vi "Measured Data (B).vi"(0 "LoadProcedure":refnum<k24>, 5 "error in (no error)":errorcluster) -> (14 "Value X":dbl[](array[numeric]), 15 "Value Y":dbl[](array[numeric]), 16 "Signal X sel":string(combo)="SetpointApplied", 17 "XY Graph":cluster{"Values":dbl[], "Values":dbl[]}(graph), 18 "Signal Y sel":string(combo)="EI_0.CalcCurrent", 19 "error out":errorcluster)   [LabVIEW 2011]
doc: "View the measured data from the procedure. The command and the command parameter of the procedure are selected with constants (basic version)."
uses:
  C:/Program Files/Metrohm Autolab/Autolab SDK 1.10/EcoChemie.Autolab.Sdk.dll
  EcoChemie.Autolab.Sdk.dll
  C:/Program Files/Metrohm Autolab/Autolab SDK 1.10/EcoChemie100.dll
  EcoChemie100.dll
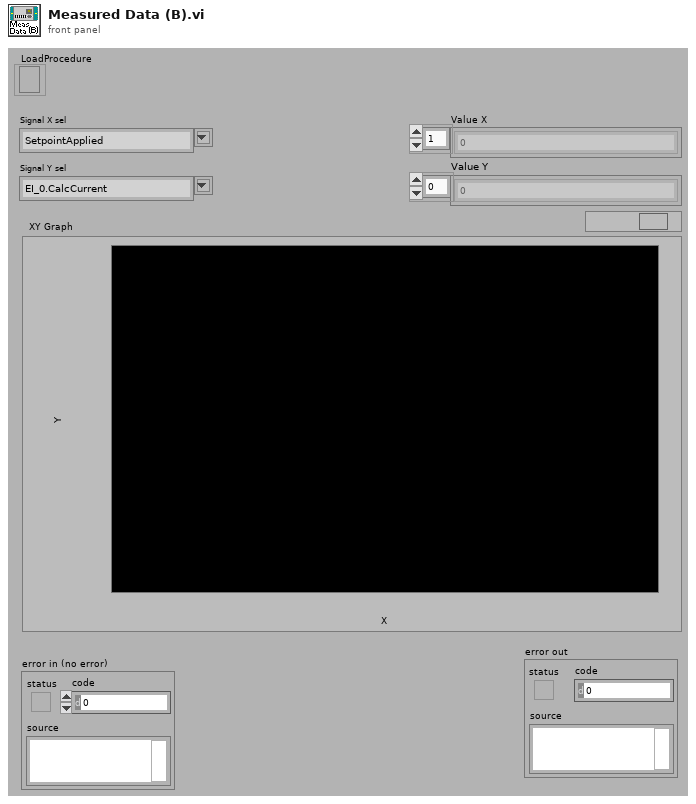
[diagram p1: front panel]
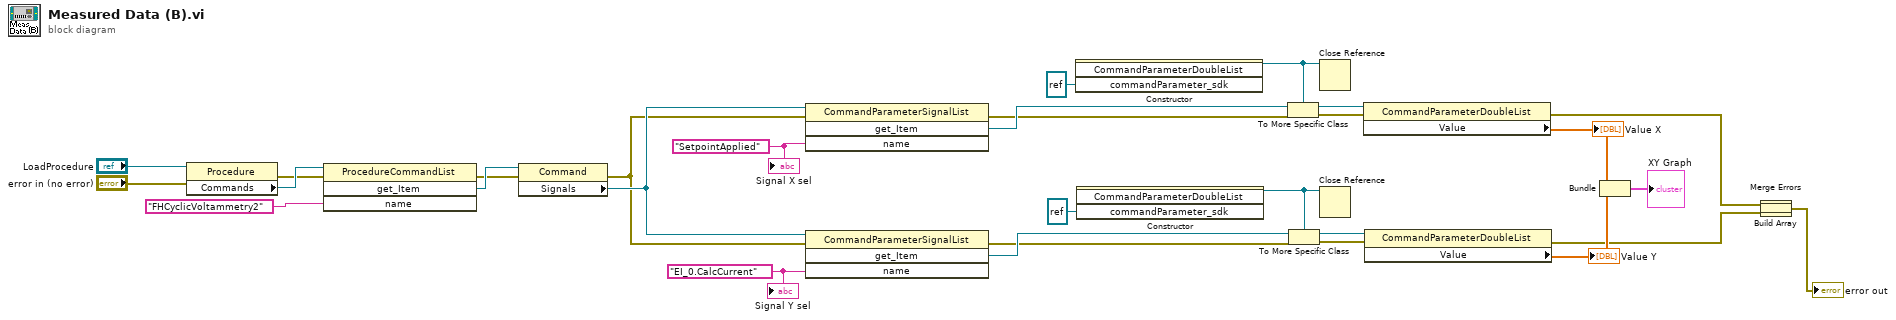
[diagram p0: block diagram]
diagram:
  w25 = "EI_0.CalcCurrent" ("Signal Y sel")
  w22 = "SetpointApplied" ("Signal X sel")
  n1 = property class="Procedure"(reference="LoadProcedure", error in="error in (no error)") -> (error out=w9:errorcluster, "Commands"=w10:refnum<k24>)  [unwired: 1 out]
  n2 = invoke class="ProcedureCommandList" method="get_Item"(reference=w10, error in=w9, "name"="FHCyclicVoltammetry2" ("ProcedureCommandList 2")) -> (error out=w6:errorcluster, "get_Item"=w7:refnum<k24>)  [unwired: 1 in, 2 out]
  n3 = property class="Command"(reference=w7, error in=w6) -> (error out=w12:errorcluster, "Signals"=w13:refnum<k24>)  [unwired: 1 out]
  n4 = invoke class="CommandParameterSignalList" method="get_Item"(reference=w13, error in=w12, "name"=w22) -> (error out=w18:errorcluster, "get_Item"=w19:refnum<k24>)  [unwired: 1 in, 2 out]
  n5 = invoke class="CommandParameterSignalList" method="get_Item"(reference=w13, error in=w12, "name"=w25) -> (error out=w20:errorcluster, "get_Item"=w21:refnum<k24>)  [unwired: 1 in, 2 out]
  n6 = constructor class="CommandParameterDoubleList"("commandParameter_sdk"=refnum<k24> refnum) -> (reference out=w5:refnum<k24>)  [unwired: 3 in, 3 out]
  n7 = constructor class="CommandParameterDoubleList"("commandParameter_sdk"=refnum<k24> refnum) -> (reference out=w4:refnum<k24>)  [unwired: 3 in, 3 out]
  n8 = To More Specific Class(target class=w5, reference=w19, error in=w18) -> (specific class reference=w15:refnum<k24>, error out=w14:errorcluster)
  n9 = To More Specific Class(target class=w4, reference=w21, error in=w20) -> (specific class reference=w17:refnum<k24>, error out=w16:errorcluster)
  n10 = Close Reference(reference=w5) -> ()  [unwired: 1 in, 1 out]
  n11 = Close Reference(reference=w4) -> ()  [unwired: 1 in, 1 out]
  n12 = property class="CommandParameterDoubleList"(reference=w15, error in=w14) -> (error out=w24:errorcluster, "Value"=w27:dbl[])  [unwired: 1 out]
  "Value X" <- w27
  n13 = property class="CommandParameterDoubleList"(reference=w17, error in=w16) -> (error out=w23:errorcluster, "Value"=w26:dbl[])  [unwired: 1 out]
  "Value Y" <- w26
  n14 = Bundle("Value"=w27, "Value"=w26) -> (→"XY Graph":cluster{"Value":dbl[], "Value":dbl[]})  [unwired: 1 in]
  n15 = Build Array(w24, w23) -> (w1:errorcluster[])
  n16 = Merge Errors(w1) -> (→"error out":errorcluster)
  "Signal X sel" <- w22
  "Signal Y sel" <- w25
